vi "lfm_rate_calculate.vi"(9 "fs":dbl=200000000.0 format="%#_13g", 10 "pw":dbl=200.0 format="%#_13g", 11 "f span":dbl) -> (3 "f skew":dbl)   [LabVIEW 2021]
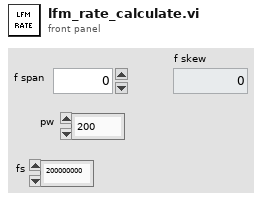
[diagram p1: front panel]
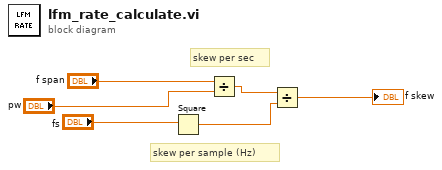
[diagram p0: block diagram]
diagram:
  # "skew per sample (Hz)"
  # "skew per sec"
  n1 = Square(x="fs") -> (x^2=w1:dbl)
  n2 = Divide(x="f span", y="pw") -> (x/y=w5:dbl)
  n3 = Divide(x=w5, y=w1) -> (x/y=→"f skew":dbl)
